vi "version_write.vi"(8 "error in (no error)":errorcluster, 10 "version":string, 11 "lv-build in":refnum<class "lv-builder-default.lvclass">) -> (0 "error out":errorcluster, 3 "lv-build out":refnum<class "lv-builder-default.lvclass">)   [LabVIEW 2015, in "lv-builder-default.lvclass"]
uses:
  lv-builder-default.lvclass
  lv-builder-default.lvclass/lv-builder-default.ctl
  lv-builder/lv-builder.lvclass
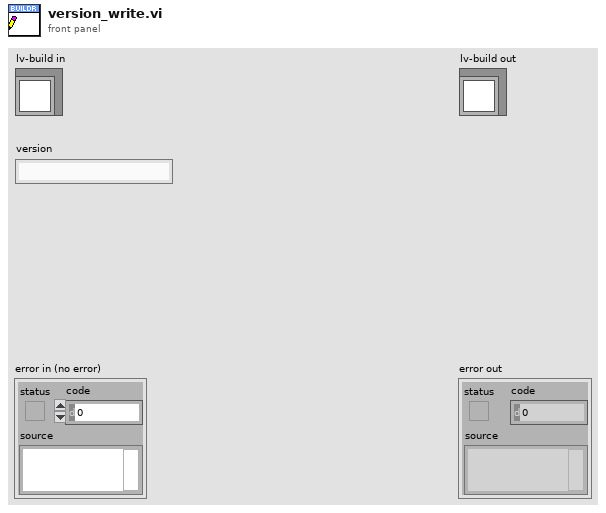
[diagram p1: front panel]
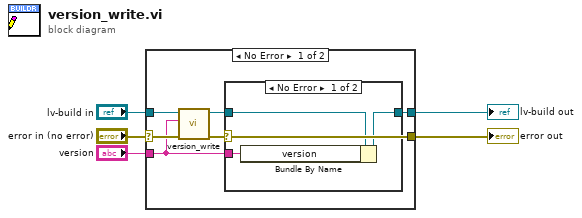
[diagram p0: block diagram]
diagram:
  n1 = case shown="No Error" "error in (no error)" {
    selector: "error in (no error)" -> [w11 w17]
    tunnel: "lv-build in" -> [w8 w16]
    tunnel: [w6 w17] -> w3
    tunnel: "version" -> [w10 _]
    tunnel: [w9 w16] -> w1
    frame No Error {
      n2 = call-parent "version_write.vi"("error in (no error)"=w11, "version"=w10, "lv-build in"=w8) -> ("error out"=w6:errorcluster, "lv-build out"=w7:refnum<class "lv-builder-default.lvclass">)  [unwired: 7 in]
      n3 = case shown="No Error" w6 {
        tunnel: w10 -> [w14 _]
        tunnel: [w13 w15] -> w9
        tunnel: w7 -> [w12 w15]
        frame No Error {
          n4 = Bundle By Name(cluster=w12, "version"=w14) -> (w13:refnum<class "lv-builder-default.lvclass">)
        }
        frame Error {
        }
      }
    }
    frame Error {
    }
  }
  "error out" <- w3
  "lv-build out" <- w1
